vi "Get Opp. Team Number.vi"(0 "DT Team":i32) -> (4 "Opp Team":i32)   [LabVIEW 2014, in "Dragon Tamers.lvlib"]
uses:
  Dragon Tamers.lvlib
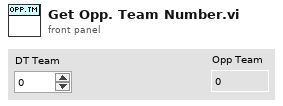
[diagram p1: front panel]
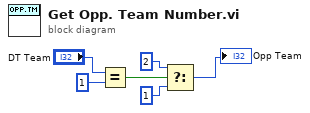
[diagram p0: block diagram]
diagram:
  n1 = Equal?(x="DT Team", y=1) -> (x = y?=w4:bool)
  n2 = Select(t=2 ("y"), s=w4, f=1 ("y")) -> (s? t:f=→"Opp Team":i32)
